vi "Normalize Coordinates.vi"(9 "Camera Type":T1, 10 "Targets":T4(array[cluster]) {"Carpet" format="%#_3g"; "Short Aspect" format="%#_3g"; "Trapezoid" format="%#_3g"; "Long Aspect" format="%#_3g"; "Area to CH" format="%#_3g"; "X Mask" format="%#_3g"; "Y Mask" format="%#_3g"}, 11 "Image in":T5) -> (2 "Found Totes":T2(array[cluster]) {"Normalized Rect"."Numeric 5" format="%#_2g"; "Normalized Rect"."Numeric 3" format="%#_2g"; "Normalized Rect"."Numeric 2" format="%#_2g"; "Normalized Rect"."Numeric" format="%#_2g"}, 3 "Sorted Scores":T3(array[cluster]) {"Carpet" format="%#_3g"; "S" format="%#_3g"; "Trapezoid %" format="%#_3g"; "L" format="%#_3g"; "Area to CH" format="%#_3g"; "X" format="%#_3g"; "Y" format="%#_3g"})   [LabVIEW 2014]
doc: "Normalize the rectangle and center so that they range from -1 to 1, left to right and bottom to top. This helps with producing joystick coordinates for driving the robot."
uses:
  <vilib>/vision/Image Controls.llb/IMAQ Image.ctl
  Camera Types.ctl
panel:
  # "Aspect Ratio"
  # "Density Profile"
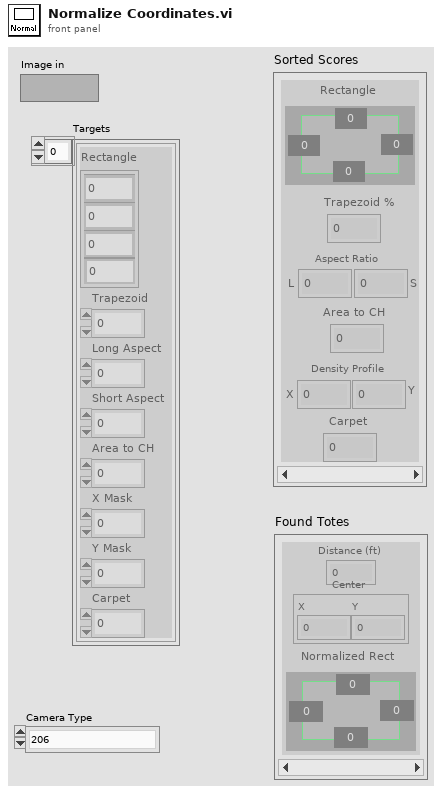
[diagram p1: front panel]
types:
  T1 = typedef "Camera Types.ctl" = enum16{"206", "1011", "1013", "MS HD3000 square", "MS HD3000 640x480"}
  T2 = cluster{"Distance (ft)":dbl, "Center":cluster{"X":dbl, "Y":dbl}, "Normalized Rect":cluster{"Numeric":dbl, "Numeric 2":dbl, "Numeric 3":dbl, "Numeric 5":dbl}}[]
  T3 = cluster{"Rectangle":cluster{"Numeric":dbl, "Numeric 2":dbl, "Numeric 3":dbl, "Numeric 5":dbl}, "Trapezoid %":dbl, "L":dbl, "S":dbl, "Area to CH":dbl, "X":dbl, "Y":dbl, "Carpet":dbl}[]
  T4 = cluster{"Rectangle":cluster{"Numeric":dbl, "Numeric 2":dbl, "Numeric 3":dbl, "Numeric 5":dbl}, "Trapezoid":dbl, "Long Aspect":dbl, "Short Aspect":dbl, "Area to CH":dbl, "X Mask":dbl, "Y Mask":dbl, "Carpet":dbl}[]
  T5 = typedef "IMAQ Image.ctl" = refnum<image>
  T6 = cluster{"Numeric":dbl, "Numeric 2":dbl, "Numeric 3":dbl, "Numeric 5":dbl}
  T7 = cluster{"X Resolution":i32, i32, "X Resolution":i32, i32}
  T8 = cluster{"Distance (ft)":dbl, cluster{dbl, dbl}, cluster{dbl, dbl, dbl, dbl}}
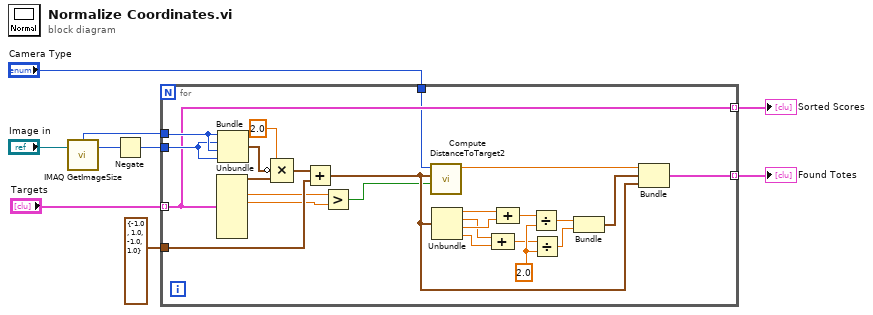
[diagram p0: block diagram]
diagram:
  n1 = call "IMAQ GetImageSize"("Image"="Image in") -> ("Y Resolution"=w7:i32, "X Resolution"=w8:i32)  [unwired: 3 in, 1 out]
  n2 = Negate(x=w7) -> (-x=w9:i32)
  n3 = for {
    tunnel: "Targets" -> [w15] mode=indexing
    tunnel: w9 -> [w33]
    tunnel: w8 -> [w34]
    tunnel: [w19] -> w4 mode=indexing
    tunnel: [w15] -> w1 mode=indexing
    tunnel: cluster{dbl, dbl, dbl, dbl} {-1.0, 1.0, -1.0, 1.0} ("y") -> [w14]
    tunnel: "Camera Type" -> [w13]
    w24 = 2.0
    n4 = Unbundle(w15) -> ("Rectangle"=w31:T6, "Long Aspect"=w12:dbl, "Short Aspect"=w11:dbl)  [unwired: 5 out]
    n5 = Bundle("X Resolution"=w34, w33, "X Resolution"=w34, w33) -> (w32:T7)  [unwired: 1 in]
    n6 = Compound Arithmetic op=MULTIPLY(2.0, invert w32, w31) -> (w30:cluster{dbl, dbl, dbl, dbl})
    n7 = Add(x=w30, y=w14) -> (x+y=w18:cluster{dbl, dbl, dbl, dbl})
    n8 = Greater?(x=w12, y=w11) -> (0:w10:bool)
    n9 = call "Compute DistanceToTarget2.vi"("Long"=w10, "Norm Rect"=w18, "Camera Type"=w13) -> ("Distance (ft)"=w17:dbl)  [unwired: 8 in]
    n10 = Unbundle(w18) -> (w28:dbl, w25:dbl, w27:dbl, w26:dbl)
    n11 = Compound Arithmetic op=ADD(w25, w26) -> (w22:dbl)
    n12 = Compound Arithmetic op=ADD(w28, w27) -> (w23:dbl)
    n13 = Divide(x=w23, y=w24) -> (x/y=w21:dbl)
    n14 = Divide(x=w22, y=w24) -> (x/y=w20:dbl)
    n15 = Bundle(w21, w20) -> (w16:cluster{dbl, dbl})  [unwired: 1 in]
    n16 = Bundle("Distance (ft)"=w17, w16, w18) -> (w19:T8)  [unwired: 1 in]
  }
  "Sorted Scores" <- w1
  "Found Totes" <- w4
